vi "xml2cluster.vi"(8 "error in":errorcluster, 10 "TypeDesc":variant, 11 "XML File Path":path) -> (0 "error out":errorcluster, 1 "XML String Out":string, 2 "data":variant)   [LabVIEW 2013]
uses:
  <vilib>/NI/GXML/_subVIs/GXML Quick Parser/Quick Parser.vi
  <vilib>/NI/GXML/GXML.lvlib
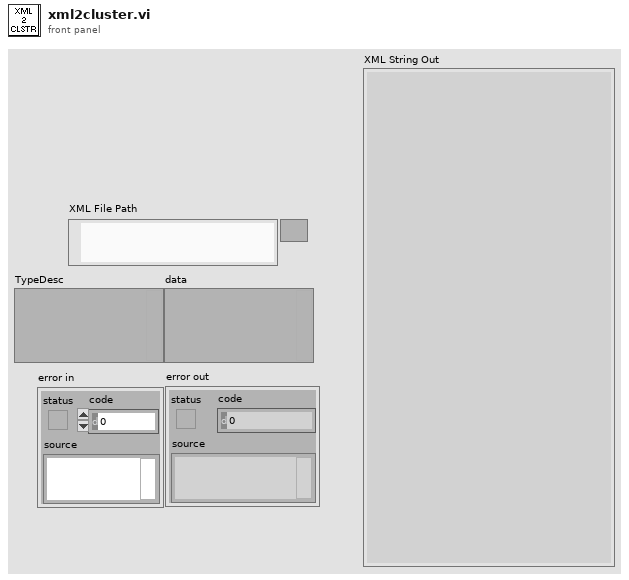
[diagram p1: front panel]
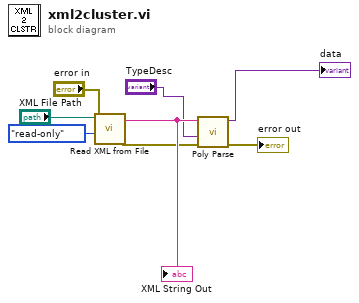
[diagram p0: block diagram]
diagram:
  n1 = call <vilib>:"Read XML from File.vi"("error in"="error in", "file access"=enum16{"read/write", "read-only", "write-only"}."read-only", "XML File Path"="XML File Path") -> ("error out"=w4:errorcluster, "XML String Out"=w5:string)  [unwired: 7 in]
  "XML String Out" <- w5
  n2 = call-poly <vilib>:"Poly Parse.vi"("error in"=w4, "TypeDesc"="TypeDesc", "XML File String"=w5) -> ("error out"=→"error out":errorcluster, "Parsed Data"=→"data":variant)  [unwired: 7 in]
